vi "TherapyBurst.vi"(0 "Input Cluster":T2 {"Therapy amplitude (mV)" format="%.2f"; "Therapy frequency (MHz)" format="%.2f"}, 1 "VISA session in":refnum<visa-resource-name>, 2 "33250(T)/33120(F)":bool, 3 "error in (no error)":errorcluster, 4 "Trigger (F) Gate(T)":bool) -> (5 "VISA session out":refnum<visa-resource-name>, 6 "Output Cluster":T1 {"Therapy amplitude (mV)" format="%.2f"; "Therapy frequency (mHz)" format="%.2f"}, 8 "error out":errorcluster)   [LabVIEW 2022 SP3]
uses:
  Pulsers/PulserGlobals.vi
panel:
  out "read buffer":string
  # "Set up to work with HP33120A. It is used as a burst source with\neither a gated burst or a fixed number of cycels"
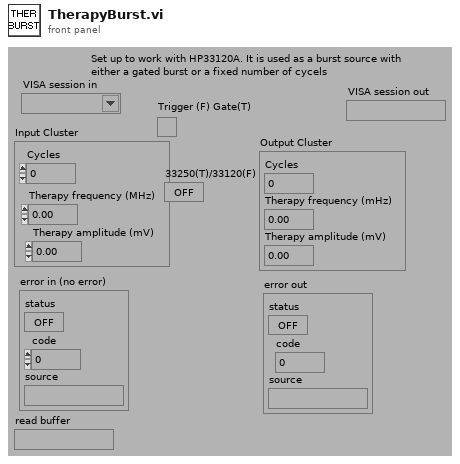
[diagram p1: front panel]
types:
  T1 = cluster{"Cycles":i32, "Therapy frequency (mHz)":dbl, "Therapy amplitude (mV)":dbl}
  T2 = cluster{"Cycles":i32, "Therapy frequency (MHz)":dbl, "Therapy amplitude (mV)":dbl}
  T3 = cluster{"Therapy frequency (MHz)":dbl, "Therapy amplitude (mV)":dbl, "time therapy on (s)":dbl, "Therapy Delay (ms) ":dbl, "Time (s)":dbl}
  T4 = cluster{"time therapy on (s)":dbl, "Therapy frequency (MHz)":dbl, "Therapy amplitude (mV)":dbl}
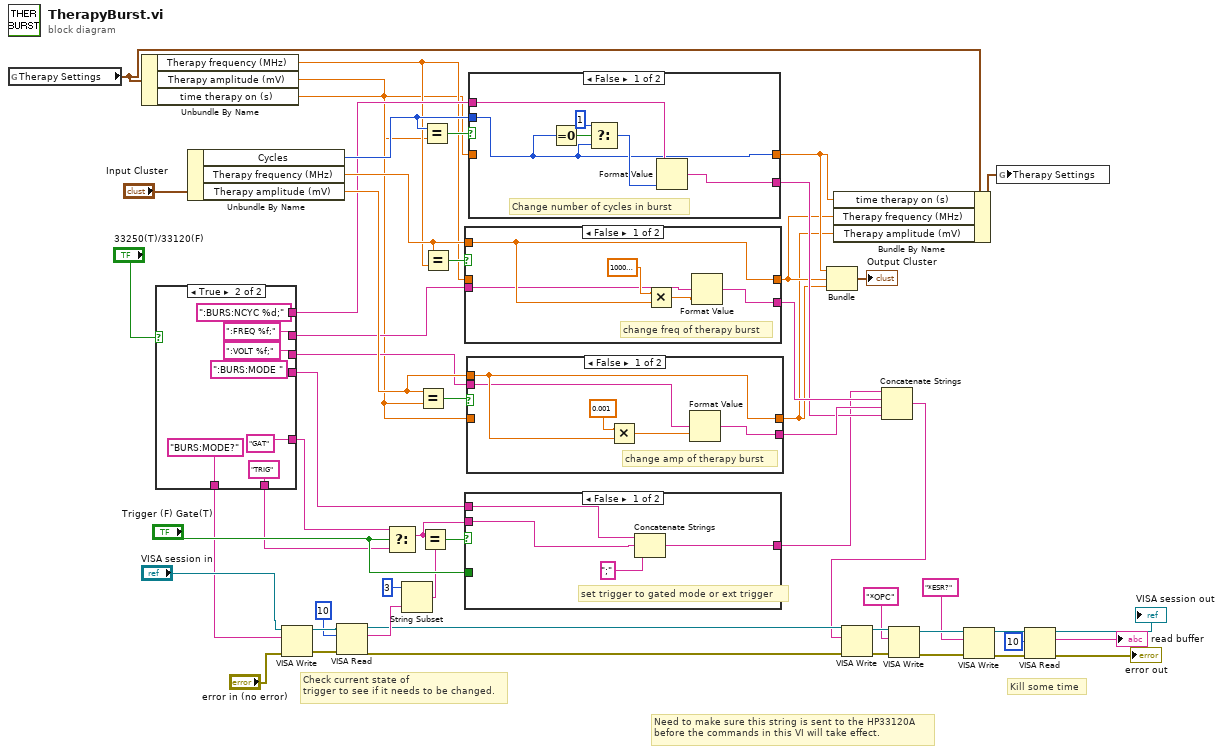
[diagram p0: block diagram]
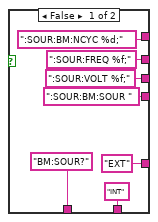
[diagram p2: hidden frame]
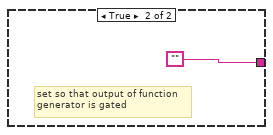
[diagram p3: hidden frame]
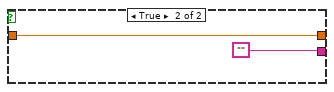
[diagram p4: hidden frame]
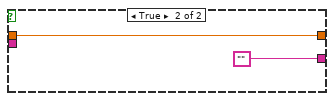
[diagram p5: hidden frame]
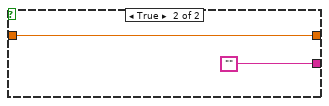
[diagram p6: hidden frame]
diagram:
  # "Kill some time"
  # "Need to make sure this string is sent to the HP33120A\nbefore the commands in this VI will take effect."
  # "Check current state of\ntrigger to see if it needs to be changed."
  n1 = global read "PulserGlobals.vi" "Therapy Settings"() -> (w5:T3)
  n2 = Unbundle By Name(w5) -> ("Therapy frequency (MHz)"=w8:dbl, "Therapy amplitude (mV)"=w7:dbl, "time therapy on (s)"=w6:dbl)
  n3 = case shown="True" "33250(T)/33120(F)" {
    tunnel: [":SOUR:BM:NCYC %d;" ":BURS:NCYC %d;"] -> w27
    tunnel: [":SOUR:FREQ %f;" ":FREQ %f;"] -> w26
    tunnel: [":SOUR:VOLT %f;" ":VOLT %f;"] -> w25
    tunnel: [":SOUR:BM:SOUR " ":BURS:MODE "] -> w24
    tunnel: ["BM:SOUR?" "BURS:MODE?"] -> w23
    tunnel: ["EXT" "GAT"] -> w22
    tunnel: ["INT" "TRIG"] -> w21
    frame False {
    }
    frame True {
    }
  }
  n4 = Unbundle By Name("Input Cluster") -> ("Cycles"=w51:i32, "Therapy frequency (MHz)"=w50:dbl, "Therapy amplitude (mV)"=w48:dbl)
  n5 = VISA Write(VISA resource name="VISA session in", write buffer=w23, error in (no error)="error in (no error)") -> (VISA resource name out=w46:refnum<visa-resource-name>, error out=w45:errorcluster)  [unwired: 1 out]
  n6 = VISA Read(VISA resource name=w46, byte count=10, error in (no error)=w45) -> (VISA resource name out=w34:refnum<visa-resource-name>, read buffer=w40:string, error out=w32:errorcluster)  [unwired: 1 out]
  n7 = Select(t=w22, s="Trigger (F) Gate(T)", f=w21) -> (s? t:f=w41:string)
  n8 = String Subset(string=w40, length (rest)=3 ("length")) -> (substring=w38:string)  [unwired: 1 out]
  n9 = Equal?(x=w48, y=w7) -> (x = y?=w49:bool)
  n10 = Equal?(x=w41, y=w38) -> (x = y?=w42:bool)
  n11 = Equal?(x=w51, y=w6) -> (x = y?=w54:bool)
  n12 = Equal?(x=w50, y=w8) -> (x = y?=w53:bool)
  n13 = case shown="False" w53 {
    tunnel: [w73 w75] -> w3
    tunnel: w8 -> [_ w75]
    tunnel: w50 -> [w73 _]
    tunnel: [w70 ""] -> w37
    tunnel: w26 -> [w69 _]
    frame False {
      # "change freq of therapy burst"
      n14 = Multiply(x=1000000.0, y=w73) -> (x*y=w72:dbl)
      n15 = Format Value(format string=w69, value (0)=w72) -> (output string=w70:string)  [unwired: 1 out]
    }
    frame True {
    }
  }
  n16 = case shown="False" w42 {
    tunnel: "Trigger (F) Gate(T)" -> [_ _]
    tunnel: w41 -> [w79 _]
    tunnel: [w78 ""] -> w29
    tunnel: w24 -> [w76 _]
    frame False {
      # "set trigger to gated mode or ext trigger"
      n17 = Concatenate Strings(w76, w79, ";") -> (w78:string)
    }
    frame True {
      # "set so that output of function\ngenerator is gated"
    }
  }
  n18 = case shown="False" w49 {
    tunnel: [w84 w87] -> w2
    tunnel: w7 -> [_ w87]
    tunnel: w48 -> [w84 _]
    tunnel: [w82 ""] -> w36
    tunnel: w25 -> [w81 _]
    frame False {
      # "change amp of therapy burst"
      n19 = Multiply(x=0.001, y=w84) -> (x*y=w83:dbl)
      n20 = Format Value(format string=w81, value (0)=w83) -> (output string=w82:string)  [unwired: 1 out]
    }
    frame True {
    }
  }
  n21 = case shown="False" w54 {
    tunnel: w51 -> [w89 _]
    tunnel: [w89 w95] -> w4
    tunnel: w6 -> [_ w95]
    tunnel: [w93 ""] -> w35
    tunnel: w27 -> [w92 _]
    frame False {
      # "Change number of cycles in burst"
      n22 = Equal To 0?(x=w89) -> (x = 0?=w91:bool)
      n23 = Select(t=1, s=w91, f=w89) -> (s? t:f=w90:i32)
      n24 = Format Value(format string=w92, value (0)=w90) -> (output string=w93:string)  [unwired: 1 out]
    }
    frame True {
    }
  }
  n25 = Bundle("time therapy on (s)"=w4, "Therapy frequency (MHz)"=w3, "Therapy amplitude (mV)"=w2) -> (→"Output Cluster":T4)  [unwired: 1 out]
  n26 = Bundle By Name(cluster=w5, "time therapy on (s)"=w4, "Therapy frequency (MHz)"=w3, "Therapy amplitude (mV)"=w2) -> (w1:T3)
  n27 = Concatenate Strings(w29, w37, w36, w35) -> (w33:string)
  n28 = VISA Write(VISA resource name=w34, write buffer=w33, error in (no error)=w32) -> (VISA resource name out=w17:refnum<visa-resource-name>, error out=w16:errorcluster)  [unwired: 1 out]
  n29 = VISA Write(VISA resource name=w17, write buffer="*OPC", error in (no error)=w16) -> (VISA resource name out=w15:refnum<visa-resource-name>, error out=w14:errorcluster)  [unwired: 1 out]
  n30 = VISA Write(VISA resource name=w15, write buffer="*ESR?", error in (no error)=w14) -> (VISA resource name out=w10:refnum<visa-resource-name>, error out=w9:errorcluster)  [unwired: 1 out]
  n31 = global write "PulserGlobals.vi" "Therapy Settings"(w1) -> ()
  n32 = VISA Read(VISA resource name=w10, byte count=10, error in (no error)=w9) -> (VISA resource name out=→"VISA session out":refnum<visa-resource-name>, read buffer=→"read buffer":string, error out=→"error out":errorcluster)  [unwired: 1 out]
